vi "string.vi"() -> ()   [LabVIEW 2020]
panel:
  out "Carga":string
  out "Sensor":string
  out "Actuador":string
  in  "Boolean":bool
  in  "Thermometer":dbl(slide) scale=0.0..100.0
  in  "Meter":u16(knob) scale=0.0..10.0
  out "length":i32
  out "Salida":string
  in  "Ingreso datos":bool
  in  "Indisque Nombre":string
  in  "Indique Apellidos":string
  out "Minusculas":string
  out "Mayusculas":string
  out "Subset":string
  out "String Concatenate":string
  out "Caracteres N":i32
  out "Dato b":string
  in  "Dato A":string
  # "String"
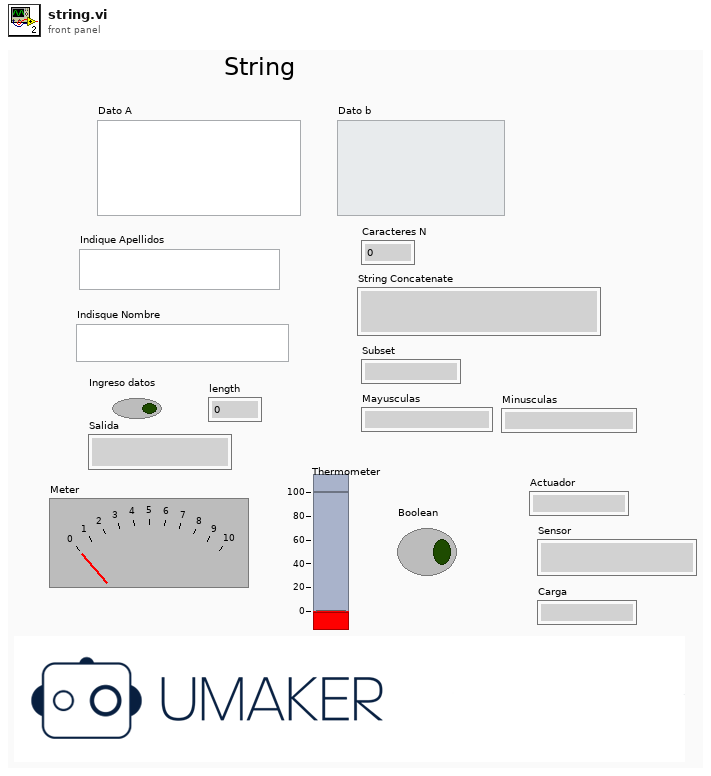
[diagram p1: front panel]
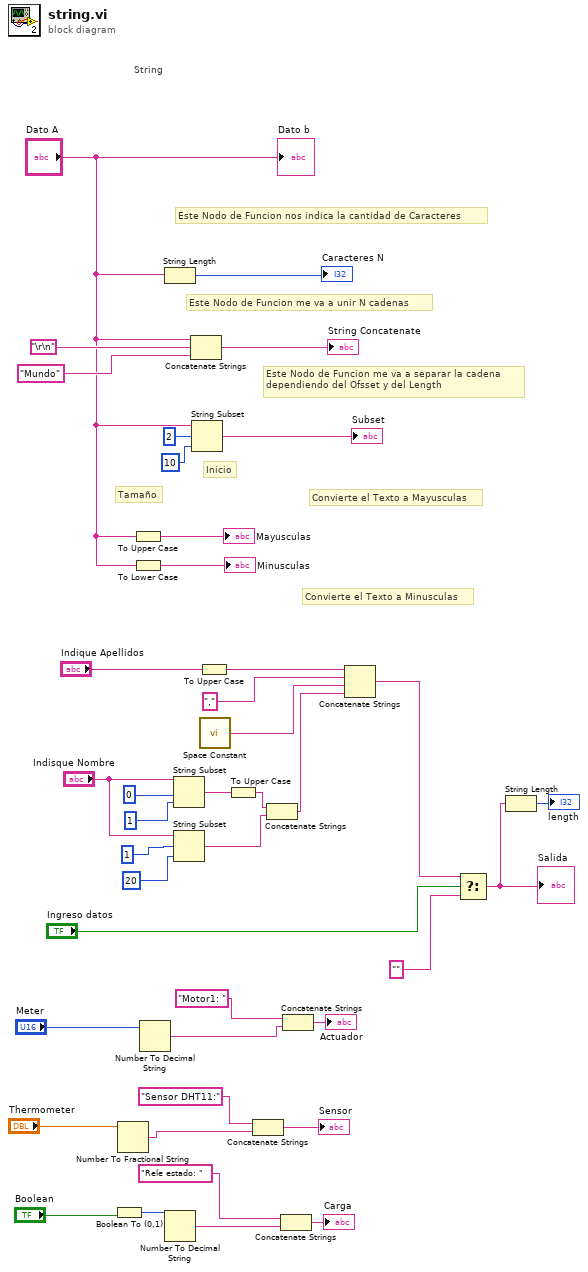
[diagram p0: block diagram]
diagram:
  # "Convierte el Texto a Minusculas"
  # "Convierte el Texto a Mayusculas"
  # "Tamaño"
  # "Inicio"
  # "Este Nodo de Funcion me va a separar la cadena \ndependiendo del Ofsset y del Length"
  # "Este Nodo de Funcion me va a unir N cadenas"
  # "Este Nodo de Funcion nos indica la cantidad de Caracteres"
  # "String"
  n1 = Boolean To (0,1)(Boolean="Boolean") -> (0, 1=w4:i16)
  n2 = Number To Fractional String(number="Thermometer") -> (F-format string=w7:string)  [unwired: 3 in]
  n3 = To Upper Case(1:"Dato A") -> (0:→"Mayusculas":string)
  n4 = To Lower Case(string="Dato A") -> (all lower case string=→"Minusculas":string)
  n5 = Number To Decimal String(number="Meter") -> (decimal integer string=w11:string)  [unwired: 1 in]
  n6 = String Length(string="Dato A") -> (length=→"Caracteres N":i32)
  n7 = Number To Decimal String(number=w4) -> (decimal integer string=w2:string)  [unwired: 1 in]
  n8 = String Subset(string="Indisque Nombre", offset (0)=0, length (rest)=1) -> (substring=w22:string)
  n9 = String Subset(string="Indisque Nombre", offset (0)=1, length (rest)=20) -> (substring=w20:string)
  n10 = Concatenate Strings("Dato A", "\r\n", "Mundo") -> (→"String Concatenate":string)
  n11 = String Subset(string="Dato A", offset (0)=2, length (rest)=10 ("length (rest)")) -> (substring=→"Subset":string)
  n12 = To Upper Case(1:"Indique Apellidos") -> (0:w30:string)
  n13 = call <vilib>:"Space Constant.vi"() -> ("String"=w28:string)
  n14 = To Upper Case(1:w22) -> (0:w21:string)
  n15 = Concatenate Strings("Sensor DHT11:", w7) -> (→"Sensor":string)
  n16 = Concatenate Strings(w21, w20) -> (w19:string)
  n17 = Concatenate Strings("Rele estado: ", w2) -> (→"Carga":string)
  n18 = Concatenate Strings("Motor1: ", w11) -> (→"Actuador":string)
  n19 = Concatenate Strings(w30, ",", w28, w19) -> (w17:string)
  n20 = Select(t=w17, s="Ingreso datos", f="") -> (s? t:f=w15:string)
  "Salida" <- w15
  n21 = String Length(string=w15) -> (length=→"length":i32)
  "Dato b" <- "Dato A"
